vi "getPictureSize.vi"(8 "error in (no error)":errorcluster, 11 "xwpfRun.Figure in":refnum<class "xwpfRun.Figure.lvclass">) -> (0 "error out":errorcluster, 3 "xwpfRun.Figure out":refnum<class "xwpfRun.Figure.lvclass">)   [LabVIEW 2017, in "Word_Specific.lvlib" / "xwpfRun.Figure.lvclass"]
uses:
  xwpfRun.Figure.lvclass
  xwpfRun.Figure.lvclass/xwpfRun.Figure.ctl
  <vilib>/picture/picture.llb/imagedata.ctl
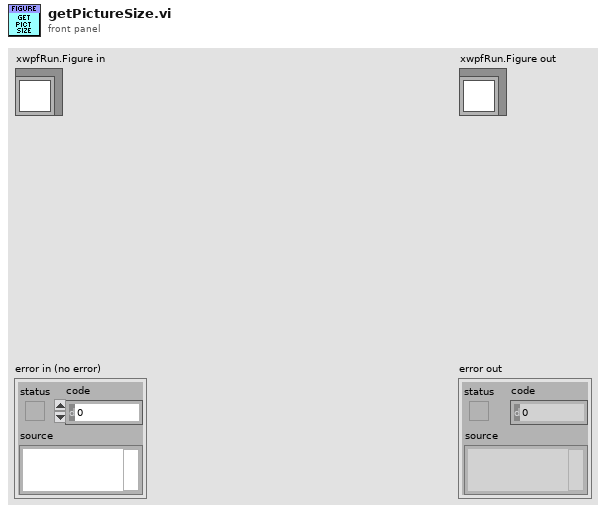
[diagram p1: front panel]
types:
  T1 = typedef "imagedata.ctl" = cluster{"image type":i32, "image depth":i32, "image":u8[], "mask":u8[], "colors":u32[], "Rectangle":cluster{"left":i16, "top":i16, "right":i16, "bottom":i16}}
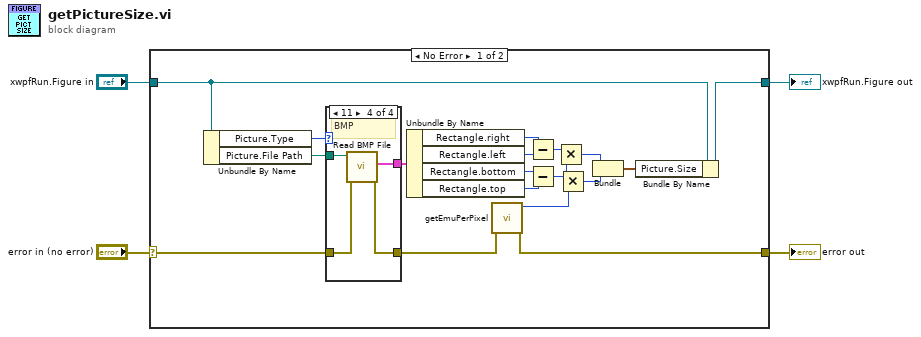
[diagram p0: block diagram]
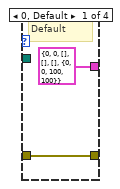
[diagram p2: hidden frame]
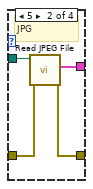
[diagram p3: hidden frame]
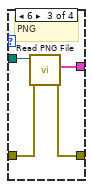
[diagram p4: hidden frame]
diagram:
  n1 = case shown="No Error" "error in (no error)" {
    selector: "error in (no error)" -> [w8 w38]
    tunnel: [w7 w38] -> w3
    tunnel: [w6 w37] -> w1
    tunnel: "xwpfRun.Figure in" -> [w12 w37]
    frame No Error {
      n2 = Unbundle By Name(w12) -> ("Picture.Type"=w11:i32, "Picture.File Path"=w10:path)
      n3 = case shown="11" w11 {
        tunnel: w10 -> [_ w28 w32 w36]
        tunnel: [T1 {"image type"=0, "image depth"=0, "image"=[], "mask"=[], "colors"=[], "Rectangle"={"left"=0, "top"=0, "right"=100, "bottom"=100}} ("image data") w27 w31 w35] -> w16
        tunnel: [w23 w26 w30 w33] -> w9
        tunnel: w8 -> [w23 w25 w29 w34]
        frame 0, Default {
          # "Default"
        }
        frame 5 {
          # "JPG"
          n4 = call <vilib>:"Read JPEG File.vi"("error in (no error)"=w25, "path to JPEG file"=w28) -> ("error out"=w26:errorcluster, "image data"=w27:T1)  [unwired: 7 in, 1 out]
        }
        frame 6 {
          # "PNG"
          n5 = call <vilib>:"Read PNG File.vi"("error in (no error)"=w29, "path to PNG file"=w32) -> ("error out"=w30:errorcluster, "image data"=w31:T1)  [unwired: 7 in, 1 out]
        }
        frame 11 {
          # "BMP"
          n6 = call <vilib>:"Read BMP File.vi"("error in (no error)"=w34, "path to BMP file"=w36) -> ("error out"=w33:errorcluster, "image data"=w35:T1)  [unwired: 7 in, 1 out]
        }
      }
      n7 = Unbundle By Name(w16) -> ("Rectangle.right"=w18:i16, "Rectangle.left"=w17:i16, "Rectangle.bottom"=w19:i16, "Rectangle.top"=w20:i16)
      n8 = call "getEmuPerPixel.vi"("error in (no error)"=w9) -> ("error out"=w7:errorcluster, "EMU_PER_PIXEL"=w13:i32)  [unwired: 9 in]
      n9 = Subtract(x=w18, y=w17) -> (x-y=w21:i16)
      n10 = Subtract(x=w19, y=w20) -> (x-y=w22:i16)
      n11 = Multiply(x=w21, y=w13) -> (x*y=w15:i32)
      n12 = Multiply(x=w22, y=w13) -> (x*y=w14:i32)
      n13 = Bundle(w15, w14) -> (w5:cluster{i32, i32})  [unwired: 1 in]
      n14 = Bundle By Name(cluster=w12, "Picture.Size"=w5) -> (w6:refnum<class "xwpfRun.Figure.lvclass">)
    }
    frame Error {
    }
  }
  "error out" <- w3
  "xwpfRun.Figure out" <- w1
